vi "设置选择.vi"(1 "设置按钮":bool) -> (0 "rate":dbl=1000.0 caption="采样速率" format="%0.2f", 2 "number of samples per channel":i32=1000 caption="每通道采样数", 3 "传感器灵敏度":dbl=200.0, 4 "主轴转速":dbl=200.0, 5 "采样时间":dbl=200.0, 6 "轴与传感器间的阈值距离":dbl=1000.0 caption="传感器与轴的阈值距离")   [LabVIEW 2014]
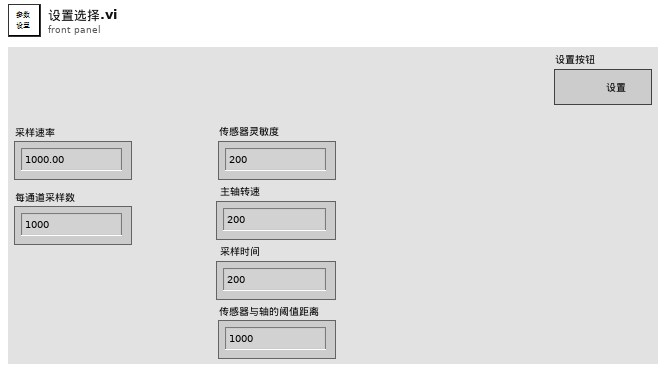
[diagram p1: front panel]
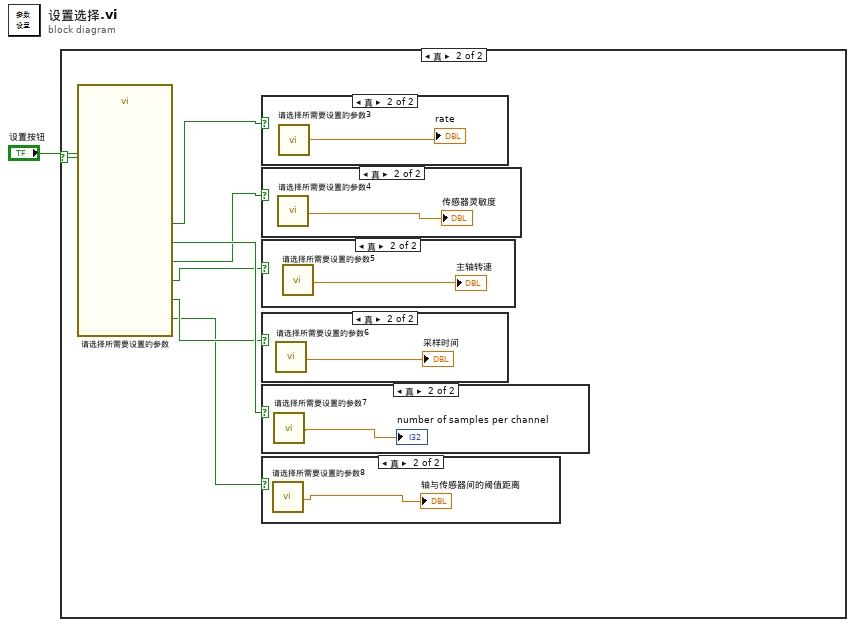
[diagram p0: block diagram]
diagram:
  n1 = case shown="真" "设置按钮" {
    frame False {
    }
    frame True {
      n2 = call "请选择所需要设置的参数"() -> ("轴与传感器间的阈值距离（μm）"=w2:bool, "采样时间（s）"=w3:bool, "主轴转速（r/min）"=w4:bool, "传感器灵敏度（μm/v）"=w5:bool, "样本大小"=w6:bool, "采样频率"=w7:bool)  [unwired: 12 in, 2 out]
      n3 = case shown="真" w7 {
        frame False {
        }
        frame True {
          n4 = call "请选择所需要设置的参数3"() -> ("采样频率"=→"rate":dbl)  [unwired: 17 in, 2 out]
        }
      }
      n5 = case shown="真" w5 {
        frame False {
        }
        frame True {
          n6 = call "请选择所需要设置的参数4"() -> ("传感器灵敏度（μm/v）"=→"传感器灵敏度":dbl)  [unwired: 17 in, 2 out]
        }
      }
      n7 = case shown="真" w4 {
        frame False {
        }
        frame True {
          n8 = call "请选择所需要设置的参数5"() -> ("主轴转速（r/min）"=→"主轴转速":dbl)  [unwired: 17 in, 2 out]
        }
      }
      n9 = case shown="真" w3 {
        frame False {
        }
        frame True {
          n10 = call "请选择所需要设置的参数6"() -> ("采样时间（s）"=→"采样时间":dbl)  [unwired: 17 in, 2 out]
        }
      }
      n11 = case shown="真" w6 {
        frame False {
        }
        frame True {
          n12 = call "请选择所需要设置的参数7"() -> ("样本大小"=→"number of samples per channel":dbl)  [unwired: 17 in, 2 out]
        }
      }
      n13 = case shown="真" w2 {
        frame False {
        }
        frame True {
          n14 = call "请选择所需要设置的参数8"() -> ("轴与传感器间的阈值距离（μm）"=→"轴与传感器间的阈值距离":dbl)  [unwired: 17 in, 2 out]
        }
      }
    }
  }
